vi "_PC_Daemon_Laser_Setting.vi"(2 "error in (no error)":errorcluster, 3 "Data":variant) -> (0 "error out":errorcluster, 1 "LaserSetting":T1={"Energy"=50.0, "Freq"=100.0, "Emission"=FALSE, "TriggerSource"=enum."Internal", "Time Stamp"=timestamp(0 s since 1904-01-01)})   [LabVIEW 2018]
uses:
  RT/ControlLoop/Laser/Ctl/_ctl_LaserParam.ctl
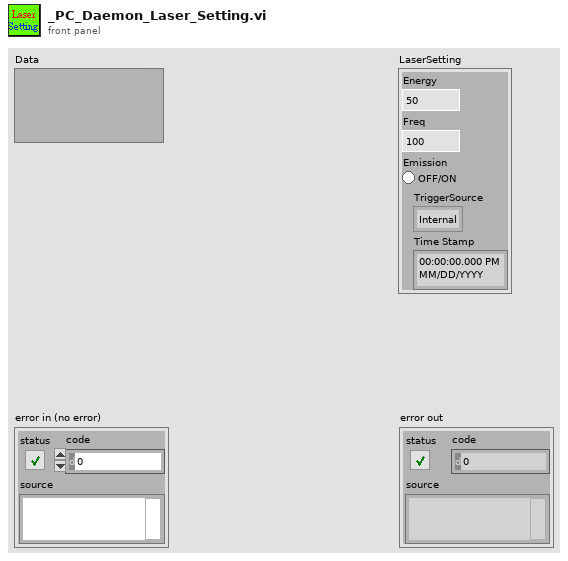
[diagram p1: front panel]
types:
  T1 = typedef "_ctl_LaserParam.ctl" = cluster{"Energy":dbl, "Freq":dbl, "Emission":bool, "TriggerSource":enum16{"Internal", "External"}, "Time Stamp":timestamp}
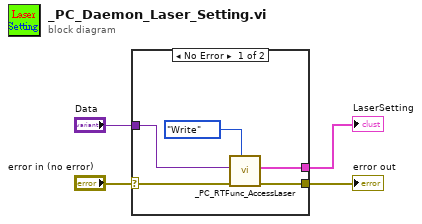
[diagram p0: block diagram]
diagram:
  n1 = case shown="No Error" "error in (no error)" {
    selector: "error in (no error)" -> [w8 w10]
    tunnel: "Data" -> [w9 _]
    tunnel: [w7 w10] -> w1
    tunnel: [w6 _] -> w2
    frame No Error {
      n2 = call "_PC_RTFunc_AccessLaser.vi"("Function"=enum16{"Init", "Write", "Read"}."Write", "error in (no error)"=w8, "Data"=w9) -> ("error out"=w7:errorcluster, "LaserSetting"=w6:T1)  [unwired: 7 in]
    }
    frame Error {
    }
  }
  "error out" <- w1
  "LaserSetting" <- w2
